vi "HideIndicators.vi"(6 "Str Refnum":refnum<vi>, 9 "DigNum Refnum 3":refnum<vi>, 10 "DigNum Refnum in":refnum<vi>, 11 "Digital in":refnum<vi>) -> ()   [LabVIEW 2021]
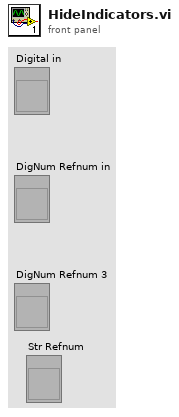
[diagram p1: front panel]
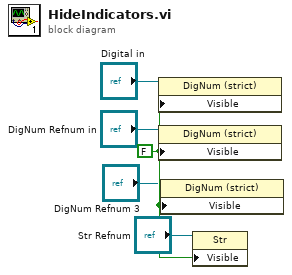
[diagram p0: block diagram]
diagram:
  w5 = FALSE ("Visible")
  n1 = property on="Property Node" class="DigNum (strict)"(reference="Digital in", "Visible"=w5) -> ()  [unwired: 1 in, 2 out]
  n2 = property on="Property Node" class="DigNum (strict)"(reference="DigNum Refnum in", "Visible"=w5) -> ()  [unwired: 1 in, 2 out]
  n3 = property on="Property Node" class="DigNum (strict)"(reference="DigNum Refnum 3", "Visible"=w5) -> ()  [unwired: 1 in, 2 out]
  n4 = property on="Property Node" class="Str"(reference="Str Refnum", "Visible"=w5) -> ()  [unwired: 1 in, 2 out]
